vi "Version not installed (no architecture available)--error.vi"(11 "Version":string) -> (0 "error out":errorcluster)   [LabVIEW 2025]
doc: "Indicates that the specified TestStand version was not found."
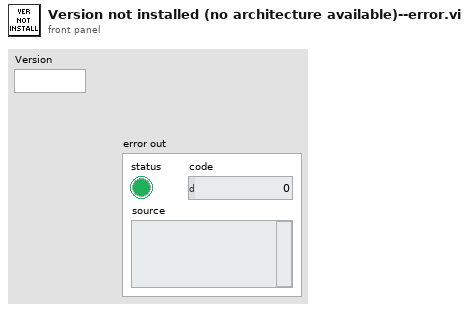
[diagram p1: front panel]
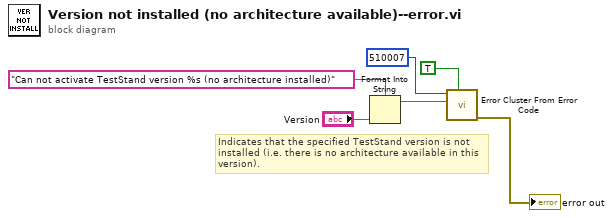
[diagram p0: block diagram]
diagram:
  # "Indicates that the specified TestStand version is not installed (i.e. there is no architecture available in this version)."
  n1 = Format Into String(format string="Can not activate TestStand version %s (no architecture installed)" ("error message (\"\")"), "Version") -> (resulting string=w1:string)  [unwired: 2 in, 1 out]
  n2 = call <vilib>:"Error Cluster From Error Code.vi"("show call chain? (False)"=TRUE, "error message (\"\")"=w1, "error code (0)"=510007) -> ("error out"=→"error out":errorcluster)  [unwired: 6 in]
